vi "Get-action-default-settings.vi"(8 "error in (no error)":errorcluster, 9 "Motor actions":T1, 10 "Action in":refnum<class "Action.lvclass">, 11 "Motor in":refnum<class "Motor.lvclass">) -> (0 "error out":errorcluster, 2 "Action":refnum<class "Action.lvclass">, 3 "Motor out":refnum<class "Motor.lvclass">)   [LabVIEW 2013, in "PowderDeposition.lvlib" / "Motor.lvclass"]
uses:
  Motor.lvclass
  Action/Motor-actions.ctl
  Action/Action.lvclass
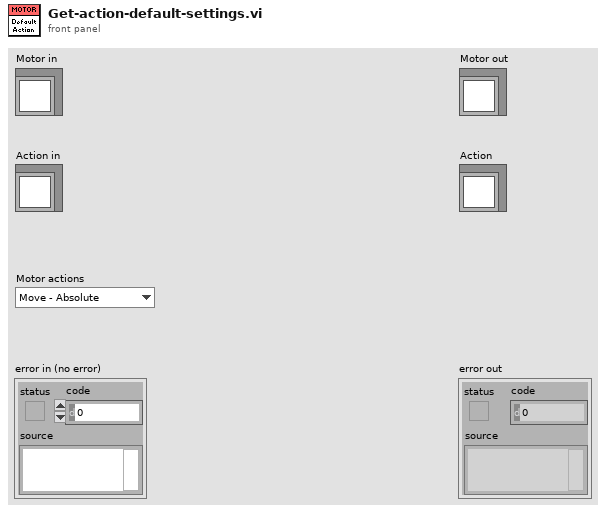
[diagram p1: front panel]
types:
  T1 = typedef "PowderDeposition.lvlib/Action.lvclass/Motor-actions.ctl" = enum16{"Move - Absolute", "Move - Relative", "Move - Timer", "Wait", "Home", "Substrate", "Sieve", "Stop"}
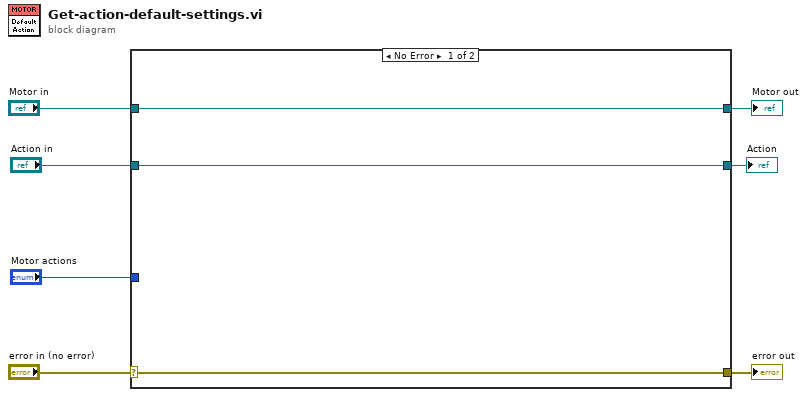
[diagram p0: block diagram]
diagram:
  n1 = case shown="No Error" "error in (no error)" {
    selector: "error in (no error)" -> [w9 w13]
    tunnel: [w9 w13] -> w6
    tunnel: [w10 w12] -> w4
    tunnel: "Motor in" -> [w10 w12]
    tunnel: "Motor actions" -> [_ _]
    tunnel: "Action in" -> [w8 w11]
    tunnel: [w8 w11] -> w1
    frame No Error {
    }
    frame Error {
    }
  }
  "error out" <- w6
  "Motor out" <- w4
  "Action" <- w1
